vi "wait_scan_start (SubVI).vi"(7 "Y (m)":sgl, 8 "error in (no error)":errorcluster, 9 "Numeric":sgl, 10 "X (m)":sgl, 11 "Application in":refnum<vi>) -> (0 "error out":errorcluster, 3 "Application out":refnum<vi>)   [LabVIEW 2014]
uses:
  <userlib>/Nanonis Prog Interface V5/Nanonis Prog Interface.lvlib
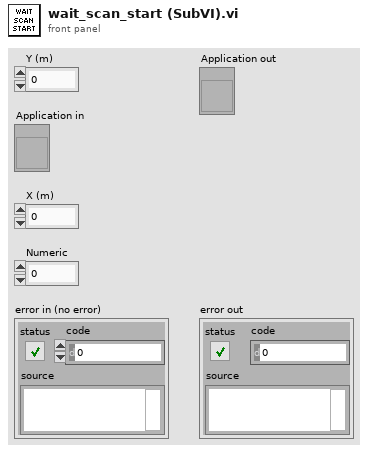
[diagram p1: front panel]
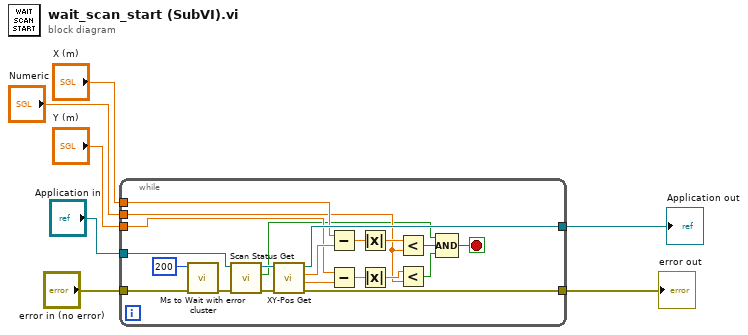
[diagram p0: block diagram]
diagram:
  n1 = while {
    tunnel: "error in (no error)" -> [w25]
    tunnel: "Application in" -> [w28]
    tunnel: [w21] -> w3
    tunnel: [w22] -> w4
    tunnel: "Y (m)" -> [w18]
    tunnel: "X (m)" -> [w17]
    tunnel: "Numeric" -> [w12]
    stop <- w9 stop-if-true
    n2 = call <userlib>:"Ms to Wait with error cluster.vi"("error in (no error)"=w25, "milliseconds to wait"=u32 200) -> ("error out"=w26:errorcluster)  [unwired: 4 in, 1 out]
    n3 = call <userlib>:"Scan Status Get.vi"("error in (no error)"=w26, "Application ref in"=w28) -> ("error out"=w24:errorcluster, "Scanning?"=w11:bool, "Application ref out"=w23:refnum<vi>)  [unwired: 6 in]
    n4 = call <userlib>:"XY-Pos Get.vi"("error in (no error)"=w24, "Application ref in"=w23) -> ("error out"=w21:errorcluster, "Y (m)"=w19:sgl, "X (m)"=w20:sgl, "Application ref out"=w22:refnum<vi>)  [unwired: 5 in]
    n5 = Subtract(x=w17, y=w20) -> (x-y=w16:sgl)
    n6 = Subtract(x=w18, y=w19) -> (x-y=w15:sgl)
    n7 = Absolute Value(x=w16) -> (abs(x)=w14:sgl)
    n8 = Absolute Value(x=w15) -> (abs(x)=w13:sgl)
    n9 = Less?(x=w14, y=w12) -> (x < y?=w8:bool)
    n10 = Less?(x=w13, y=w12) -> (x < y?=w10:bool)
    n11 = Compound Arithmetic op=AND(w11, w8, w10) -> (w9:bool)
  }
  "Application out" <- w4
  "error out" <- w3
